vi "Update Self Unified Actor.vi"(7 "Actor in":refnum<class "Actor.lvclass">, 10 "This VI":refnum<vi>) -> (0 "Error out":errorcluster, 5 "Actor out":refnum<class "Actor.lvclass">)   [LabVIEW 2020, in "jettl.lvlib"]
uses:
  jettl.lvlib
  Actor/Actor.lvclass
  Message/Message.lvclass
  ActorRelation.ctl
  MessageMetadata.ctl
  Message.ctl
  ActorLifetime.ctl
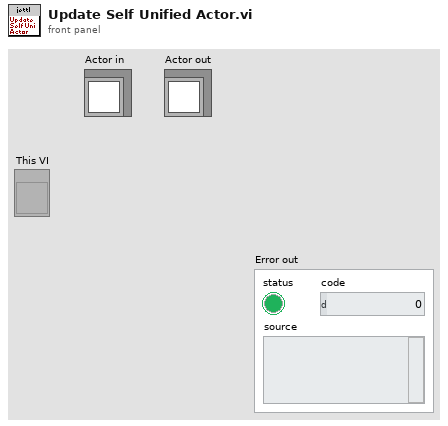
[diagram p1: front panel]
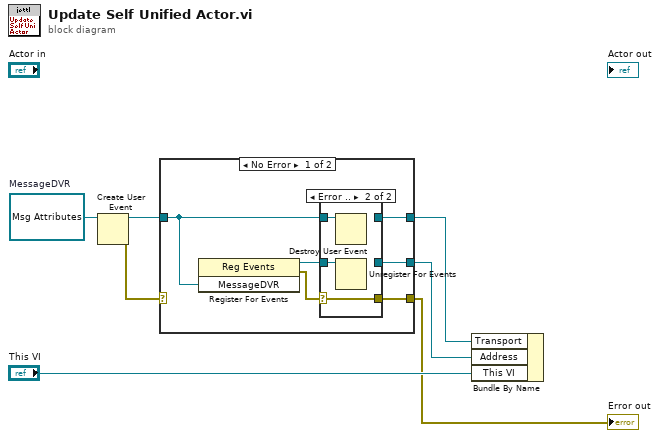
[diagram p0: block diagram]
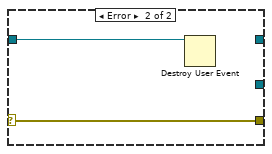
[diagram p3: hidden frame]
diagram:
  w3 = refnum<data-value> refnum  # MessageDVR
  n1 = Create User Event(user event datatype=w3) -> (user event=w7:refnum<user-event>, error out=w8:errorcluster)  [unwired: 1 in]
  n2 = case shown="No Error" w8 {
    selector: w8 -> [_ w24]
    tunnel: [w17 w24] -> w6
    tunnel: w7 -> [w12 w23]
    tunnel: [w16 _] -> w2
    tunnel: [w15 _] -> w1
    frame No Error {
      n3 = register-events(w12) -> (reference out=w13:refnum<event-registration>, error out=w14:errorcluster)  [unwired: 2 in]
      n4 = case shown="Error .." w14 {
        selector: w14 -> [_ w22]
        tunnel: [_ w22] -> w17
        tunnel: [w19 _] -> w15
        tunnel: w13 -> [w19 w21]
        tunnel: [w18 _] -> w16
        tunnel: w12 -> [w18 w20]
        frame No Error {
        }
        frame Error {
          n5 = Destroy User Event(user event=w20) -> ()  [unwired: 1 in, 1 out]
          n6 = Unregister For Events(event registration refnum=w21) -> ()  [unwired: 1 in, 1 out]
        }
      }
    }
    frame Error {
      n7 = Destroy User Event(user event=w23) -> ()  [unwired: 1 in, 1 out]
    }
  }
  "Error out" <- w6
  n8 = Bundle By Name("Transport"=w2, "Address"=w1, "This VI"="This VI") -> (w4:cluster{}, w5:cluster{})
